vi "读取-设备终端.lvclass.vi"(8 "error in (no error)":errorcluster caption="错误输入（无错误）", 11 "PC个人客户端输入":refnum<class "PC个人客户端.lvclass">) -> (0 "error out":errorcluster caption="错误输出", 2 "设备终端.lvclass":refnum<class "设备终端.lvclass">, 3 "PC个人客户端输出":refnum<class "PC个人客户端.lvclass">)   [LabVIEW 2013, in "PC个人客户端.lvclass"]
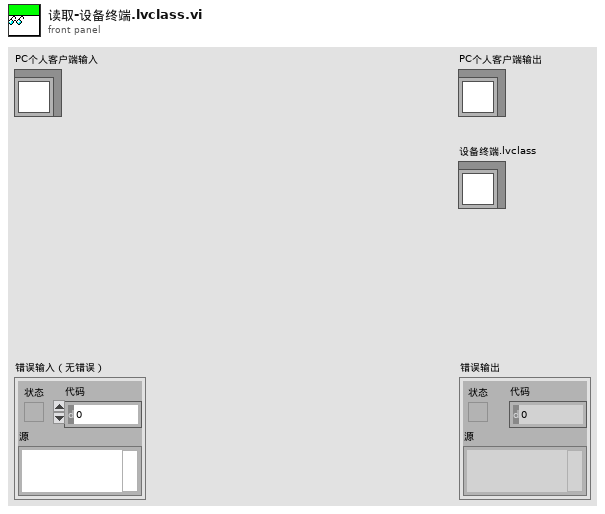
[diagram p1: front panel]
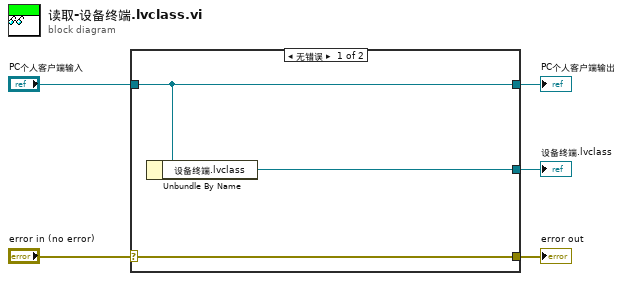
[diagram p0: block diagram]
diagram:
  n1 = case shown="无错误" "error in (no error)" {
    selector: "error in (no error)" -> [w8 w9]
    tunnel: [w8 w9] -> w4
    tunnel: [w7 w10] -> w2
    tunnel: "PC个人客户端输入" -> [w7 w10]
    tunnel: [w6 _] -> w1
    frame No Error {
      n2 = Unbundle By Name(w7) -> ("设备终端.lvclass"=w6:refnum<class "设备终端.lvclass">)
    }
    frame Error {
    }
  }
  "error out" <- w4
  "PC个人客户端输出" <- w2
  "设备终端.lvclass" <- w1
